vi "Read from Bound.vi"() -> (0 "error out":errorcluster, 3 "Bound":dbl)   [LabVIEW 2013]
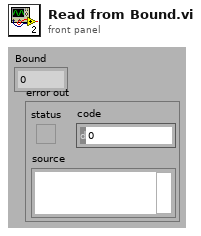
[diagram p1: front panel]
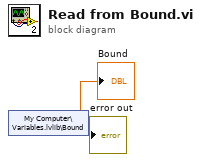
[diagram p0: block diagram]
diagram:
  n1 = shared-variable "My Computer\\Variables.lvlib\\Bound"() -> (→"Bound":dbl, error out=→"error out":errorcluster)  [unwired: 1 out]
